vi "Write Timeout Iteration.vi"(8 "error in (no error)":errorcluster, 10 "Timeout Iteration":u32, 11 "LargeScrollbar in":refnum<class "LargeScrollbar.lvclass">) -> (0 "error out":errorcluster, 3 "LargeScrollbar out":refnum<class "LargeScrollbar.lvclass">)   [LabVIEW 2015, in "LargeScrollbar.lvclass"]
doc: "<b> </b> <b> </b>\n©2016 Q Software Innovations, LLC (QSI)\nwritten by Quentin Alldredge\nproduced in LabVIEW 2015\n\nsupport@qsoftwareinnovations.com\nwww.qsoftwareinnovations.com\n\nAll rights reserved.\n\nRedistribution and use in source and binary forms, with or without modification, are permitted provided that the following conditions are met:\n\n * Redistributions of source code must retain the above copyright notice, this list of conditions and the following disclaimer.\n * Redistributions in binary form must reproduce the above copyright notice, this list of conditions and the following disclaimer in the documentation and/or other materials provided with the distribution.\n * Neither the name of Q Software Innovations, LLC. nor the names of its contributors may be used to endorse or promote products derived from this software without specific prior written permission.\n\nTHIS SOFTWARE IS PROVIDED BY THE COPYRIGHT HOLDERS AND CONTRIBUTORS \"AS IS\" AND ANY EXPRESS OR IMPLIED WARRANTIES, INCLUDING, BUT NOT LIMITED TO, THE IMPLIED WARRANTIES OF MERCHANTABILITY AND FITNESS FOR A PARTICULAR PURPOSE ARE DISCLAIMED. IN NO EVENT SHALL THE COPYRIGHT OWNER OR CONTRIBUTORS BE LIABLE FOR ANY DIRECT, INDIRECT, INCIDENTAL, SPECIAL, EXEMPLARY, OR CONSEQUENTIAL DAMAGES (INCLUDING, BUT NOT LIMITED TO, PROCUREMENT OF SUBSTITUTE GOODS OR SERVICES; LOSS OF USE, DATA, OR PROFITS; OR BUSINESS INTERRUPTION) HOWEVER CAUSED AND ON ANY THEORY OF LIABILITY, WHETHER IN CONTRACT, STRICT LIABILITY, OR TORT (INCLUDING NEGLIGENCE OR OTHERWISE) ARISING IN ANY WAY OUT OF THE USE OF THIS SOFTWARE, EVEN IF ADVISED OF THE POSSIBILITY OF SUCH DAMAGE."
uses:
  LargeScrollbar.lvclass
  LargeScrollbar.lvclass/LargeScrollbar.ctl
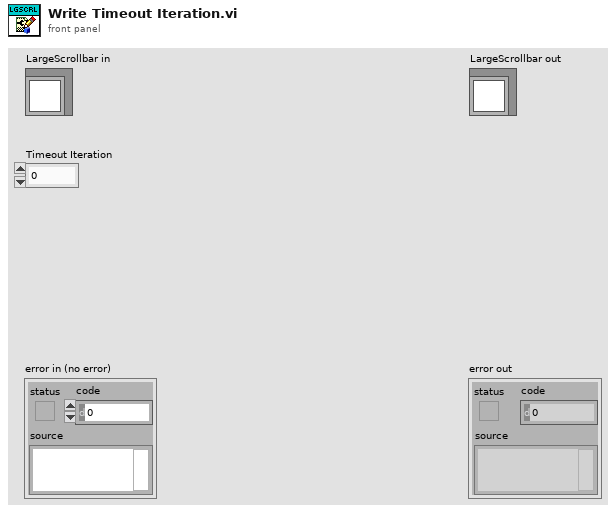
[diagram p1: front panel]
types:
  T1 = typedef "LargeScrollbar.lvclass/State Data.ctl" = cluster{"Direction":T2, "Timeout Iteration":u32}
  T2 = typedef "LargeScrollbar.lvclass/Direction.ctl" = enum16{"Decrement", "Increment"}
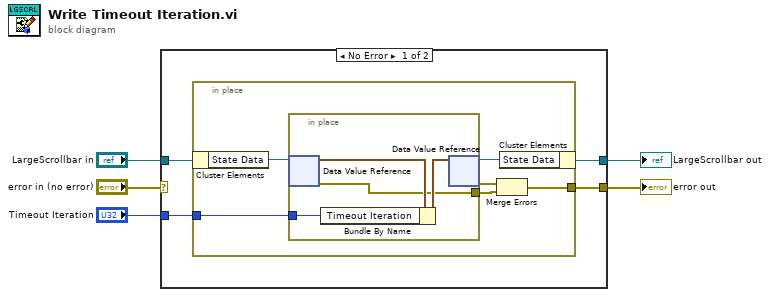
[diagram p0: block diagram]
diagram:
  n1 = case shown="No Error" "error in (no error)" {
    selector: "error in (no error)" -> [_ w21]
    tunnel: [w7 w21] -> w4
    tunnel: [w6 w20] -> w2
    tunnel: "LargeScrollbar in" -> [w9 w20]
    tunnel: "Timeout Iteration" -> [w8 _]
    frame No Error {
      n2 = in-place {
        in-place-border: w8 -> [w14]
        in-place-border: [w10] -> w7
        n3 = in-place-cluster #1(w9) -> ("State Data"=w15:refnum<data-value>)
        n4 = in-place {
          in-place-border: w14 -> [w18]
          in-place-border: [w16] -> w11
          n5 = in-place-dvr #2(w15) -> (w19:T1, w16:errorcluster)
          n6 = Bundle By Name(cluster=w19, "Timeout Iteration"=w18) -> (w17:T1)
          n7 = in-place-dvr #2(w17) -> (w13:refnum<data-value>, w12:errorcluster)
        }
        n8 = Merge Errors(w12, w11) -> (w10:errorcluster)
        n9 = in-place-cluster #1("State Data"=w13) -> (w6:refnum<class "LargeScrollbar.lvclass">)
      }
    }
    frame Error {
    }
  }
  "error out" <- w4
  "LargeScrollbar out" <- w2
